vi "Write Message Type.vi"(8 "error in (no error)":errorcluster, 10 "Message Type":variant, 11 "bt_WaitOn_Queue in":refnum<class "bt_WaitOn_Queue.lvclass">) -> (0 "error out":errorcluster, 3 "bt_WaitOn_Queue out":refnum<class "bt_WaitOn_Queue.lvclass">)   [LabVIEW 2021, in "BT.lvlib" / "bt_WaitOn_Queue.lvclass"]
uses:
  bt_WaitOn_Queue.lvclass
  bt_WaitOn_Queue.lvclass/bt_WaitOn_Queue.ctl
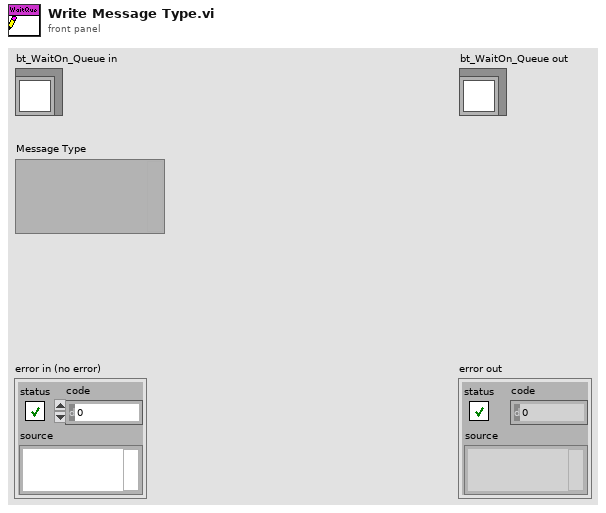
[diagram p1: front panel]
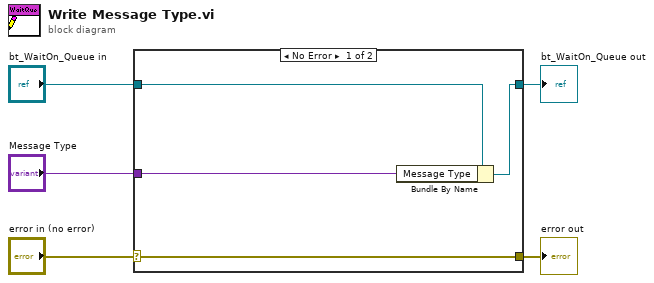
[diagram p0: block diagram]
diagram:
  n1 = case shown="No Error" "error in (no error)" {
    selector: "error in (no error)" -> [w9 w10]
    tunnel: [w9 w10] -> w4
    tunnel: [w7 w11] -> w2
    tunnel: "bt_WaitOn_Queue in" -> [w8 w11]
    tunnel: "Message Type" -> [w6 _]
    frame No Error {
      n2 = Bundle By Name(cluster=w8, "Message Type"=w6) -> (w7:refnum<class "bt_WaitOn_Queue.lvclass">)
    }
    frame Error {
    }
  }
  "error out" <- w4
  "bt_WaitOn_Queue out" <- w2
